vi "Benchmark mupLib.vi"() -> ()   [LabVIEW 2015]
panel:
  out "bulk eval time (average)":dbl format="%#_6ps"
  out "parse and eval time (average)":dbl format="%#_6ps"
  in  "Iterations":i32=10000
  out "eval time (average)":dbl format="%#_6ps"
  in  "szExpr":string="1*x^2+2*x+2"
  out "error out":errorcluster
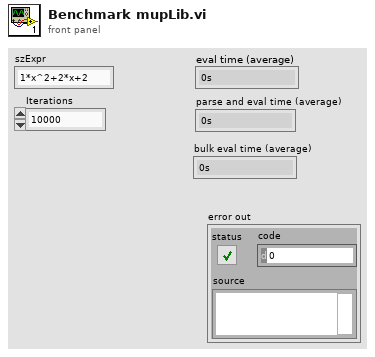
[diagram p1: front panel]
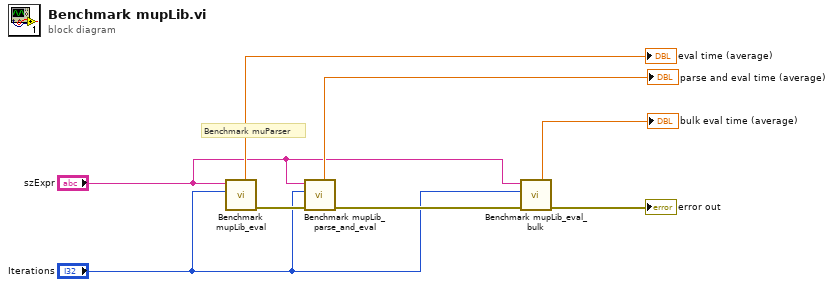
[diagram p0: block diagram]
diagram:
  # "Benchmark muParser"
  n1 = call "Benchmark mupLib_eval.vi"("Iterations"="Iterations", "Expression"="szExpr") -> ("error out"=w7:errorcluster, "dt average"=→"eval time (average)":dbl)  [unwired: 6 in, 2 out]
  n2 = call "Benchmark mupLib_parse_and_eval.vi"("error in (no error)"=w7, "Iterations"="Iterations", "Expression"="szExpr") -> ("error out"=w6:errorcluster, "dt average"=→"parse and eval time (average)":dbl)  [unwired: 5 in, 2 out]
  n3 = call "Benchmark mupLib_eval_bulk.vi"("error in (no error)"=w6, "Iterations"="Iterations", "Expression"="szExpr") -> ("error out"=→"error out":errorcluster, "dt average"=→"bulk eval time (average)":dbl)  [unwired: 5 in, 2 out]
